vi "Rotation stage shgv3.vi"() -> ()   [LabVIEW 2020]
doc: "Shows how to move a motor to an absolute position."
uses:
  <vilib>/Utility/error.llb/DialogType.ctl
  <vilib>/DAQmx/read.llb/DAQmx Read (Analog 1D Wfm NChan 1Samp).vi
  <vilib>/DAQmx/read.llb/DAQmx Read (Counter 1D U32 1Chan NSamp).vi
  <vilib>/DAQmx/create/channels.llb/DAQmx Create Channel (CI-Period).vi
  <vilib>/DAQmx/create/channels.llb/DAQmx Create Channel (CO-Pulse Generation-Frequency).vi
  <vilib>/DAQmx/configure/timing.llb/DAQmx Timing (Implicit).vi
  <vilib>/DAQmx/miscellaneous.llb/DAQmx Fill In Error Info.vi
  <vilib>/DAQmx/create/channels.llb/DAQmx Create Channel (AI-Current-Basic).vi
  <vilib>/DAQmx/configure/timing.llb/DAQmx Timing (Sample Clock).vi
  <resource>/objmgr/daqmx.rc
panel:
  out "Actual Sample Rate":dbl=1000.0 format="%0.2f"
  out "data 2":waveform(dbl)[](graph)
  out "Consumer Iteration 3":i32=1109257
  in  "stop 4":bool
  out "Producer Iteration 3":i32=1109256
  out "error out 3":errorcluster
  out "Loop Time (ms) 3":u32=10
  in  "Duty Cycle":dbl=0.5 format="%.6f"
  out "Input.BufSize":u32=1000000 format="%.0p"
  out "data":u32[](graph)
  out "Consumer Iteration 2":i32=1109257
  in  "stop 3":bool
  in  "number of samples per channel 2":i32=5000
  out "Producer Iteration 2":i32=1109256
  out "error out 2":errorcluster
  out "Loop Time (ms) 2":u32=10
  in  "dwell time (ms)":dbl=1.0 format="%.6f"
  in  "Photon Input (PFI)":tag="/Dev1/PFI0"
  in  "Rotation Angle (Degrees)":dbl=100.0 min=0.0
  in  "MG17Motor":refnum<k7>(container)
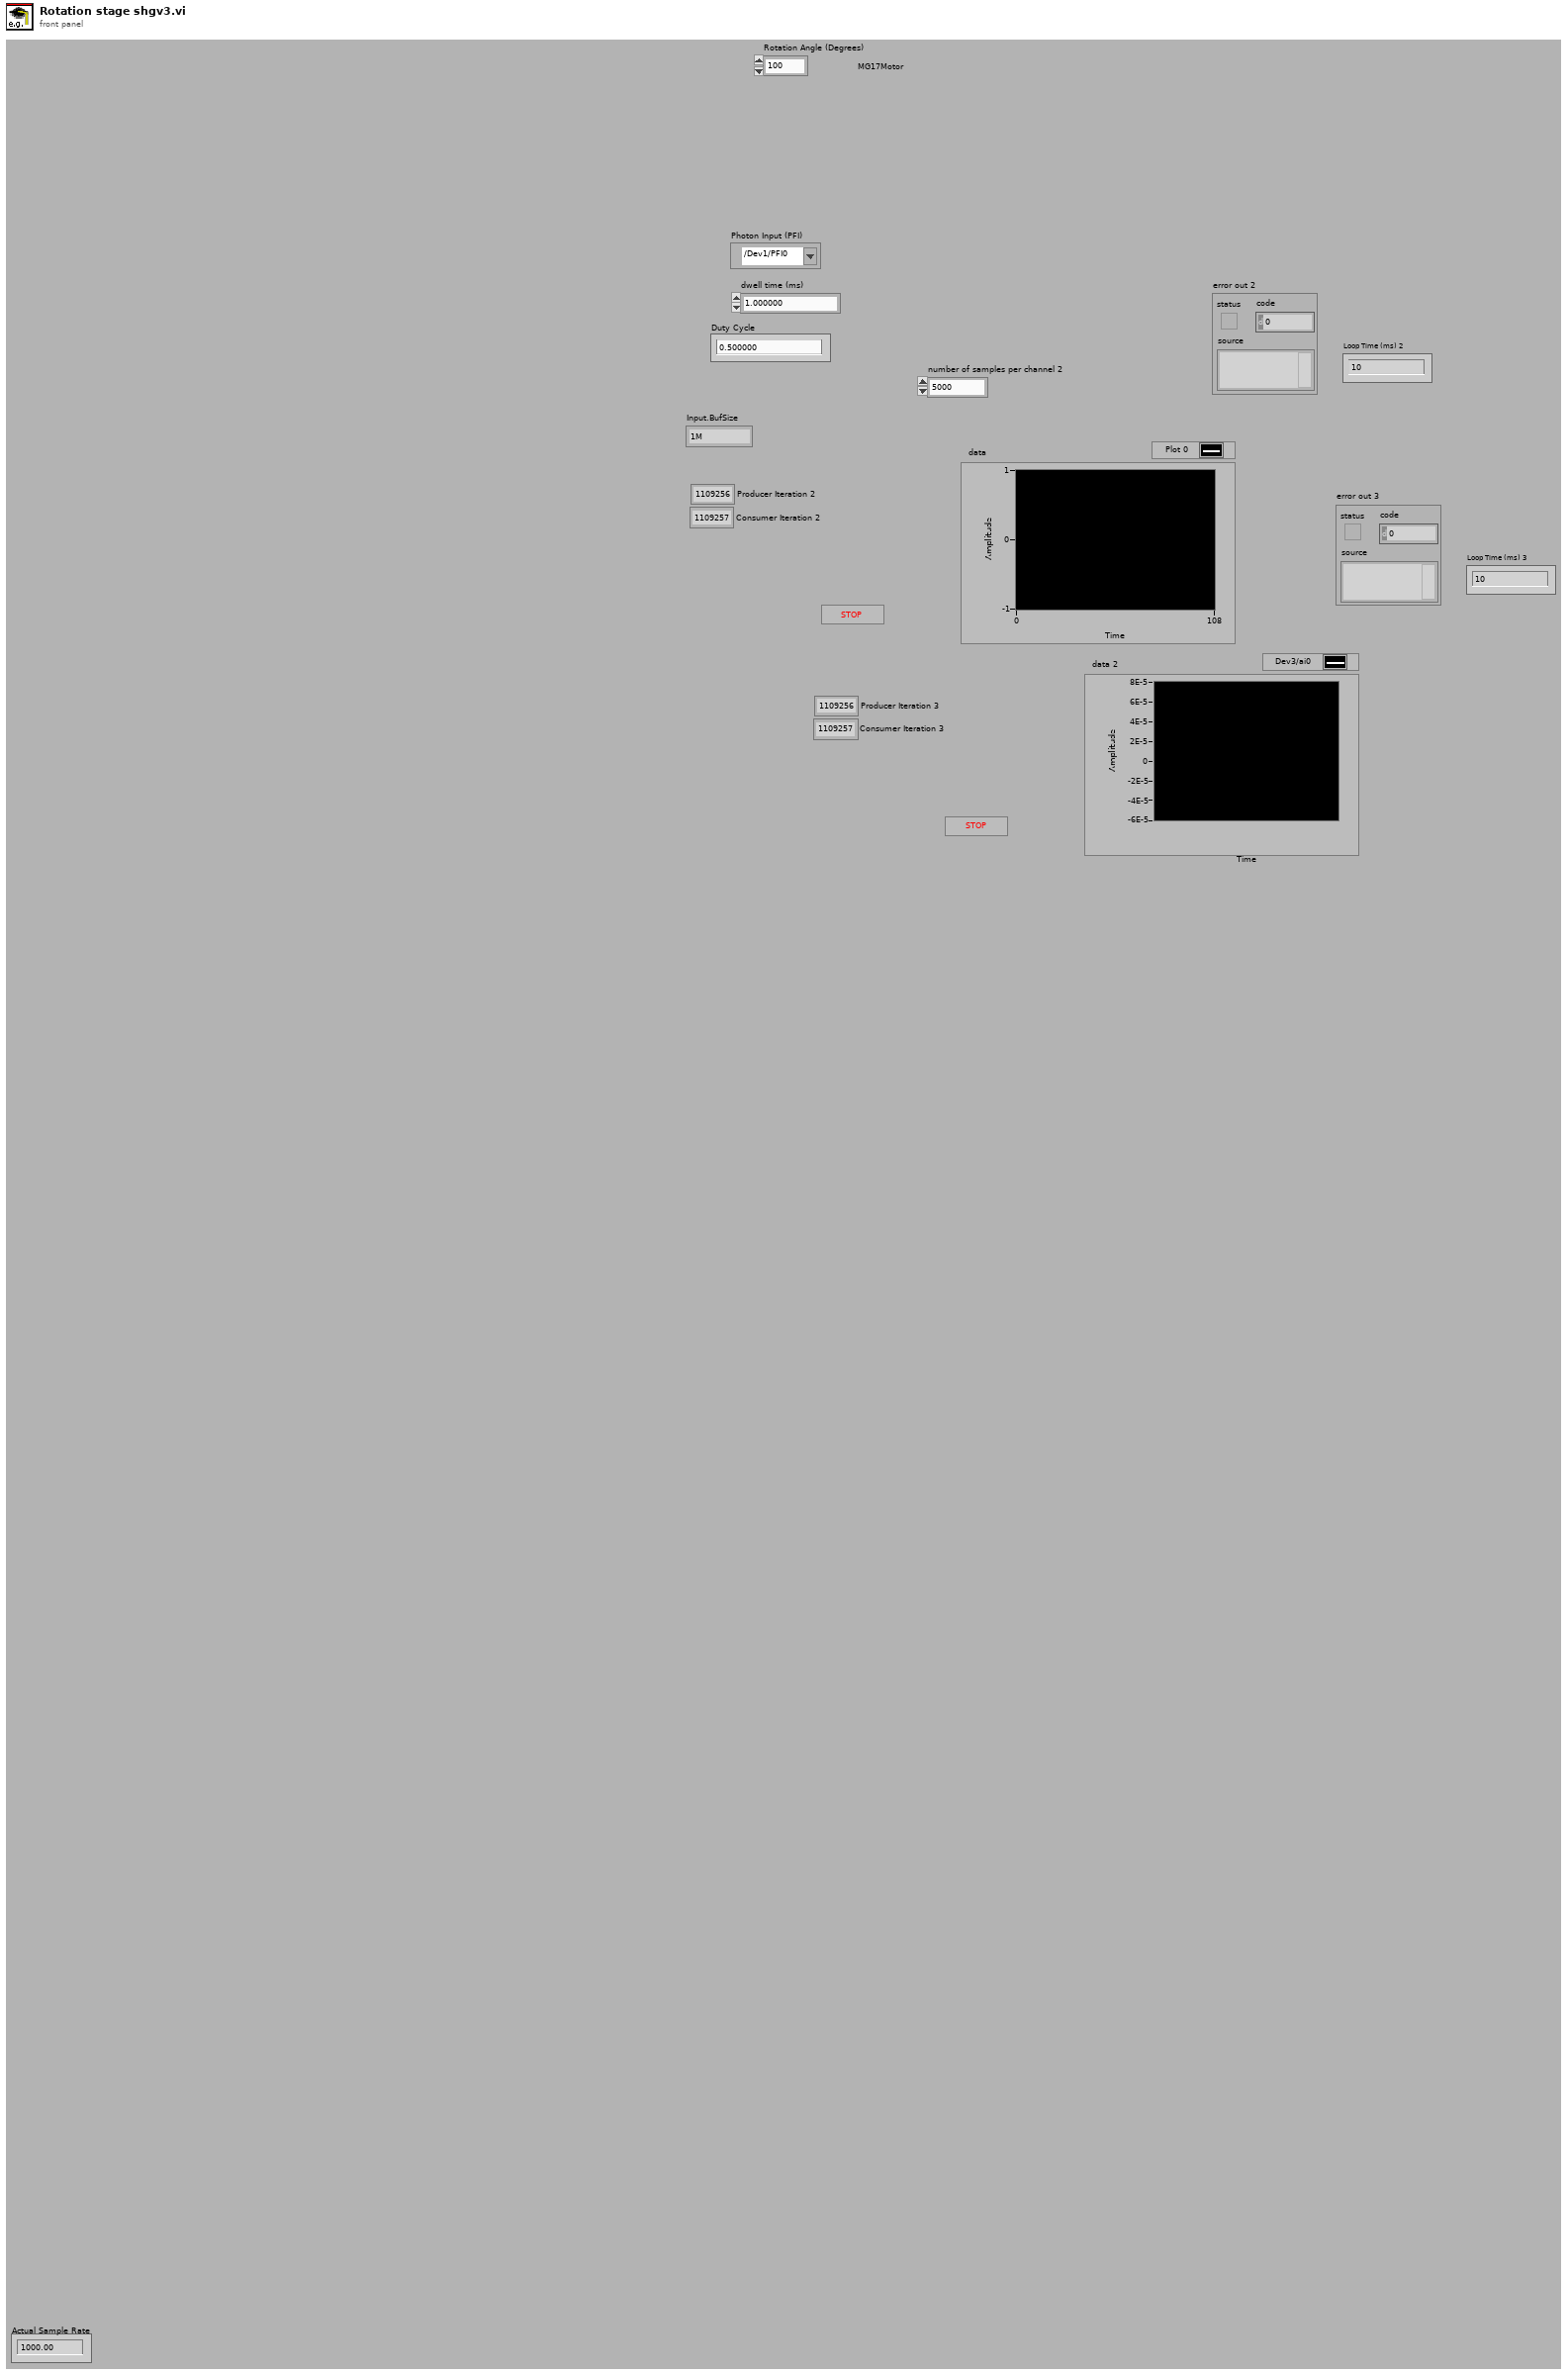
[diagram p1: front panel]
types:
  T1 = enum16{"open", "open or create", "create or replace", "create", "open (read-only)"}
  T2 = typedef "DialogType.ctl" = u16
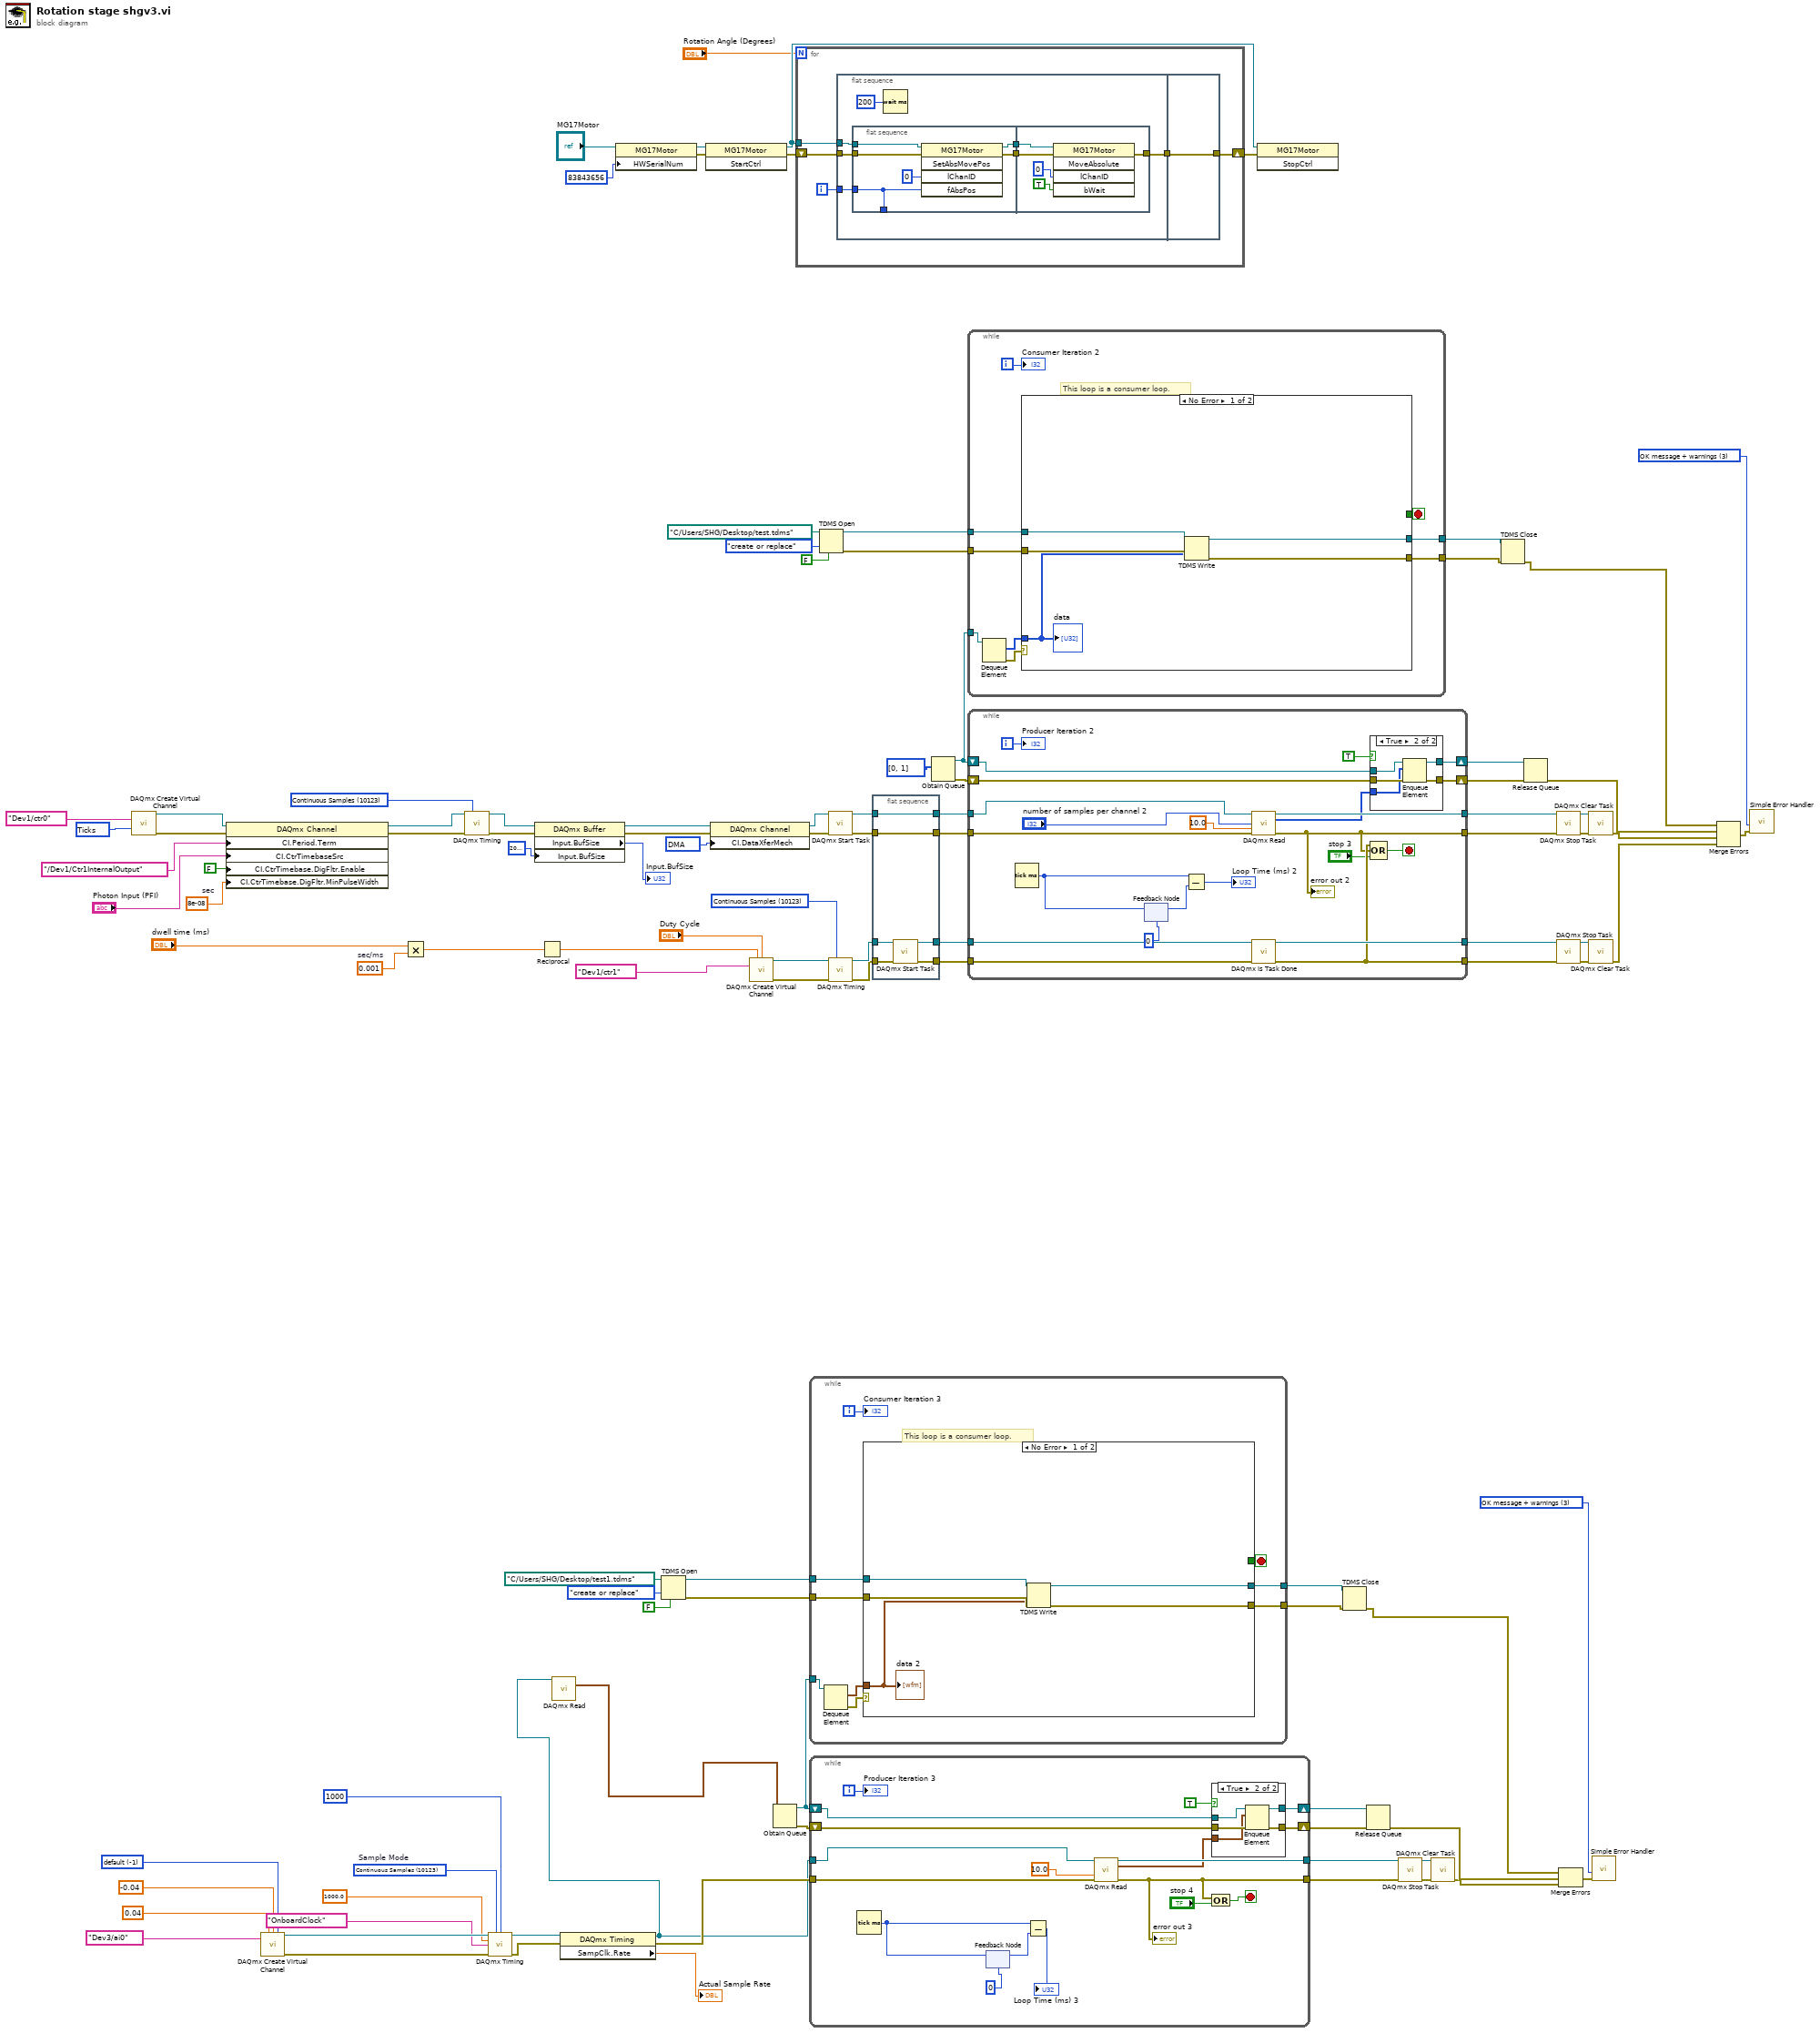
[diagram p0: block diagram]
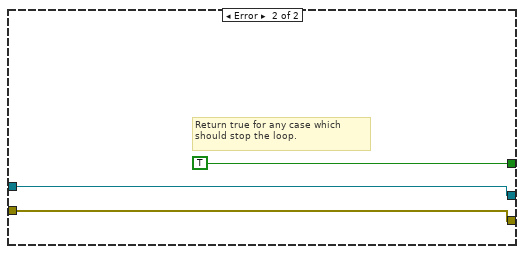
[diagram p2: hidden frame]
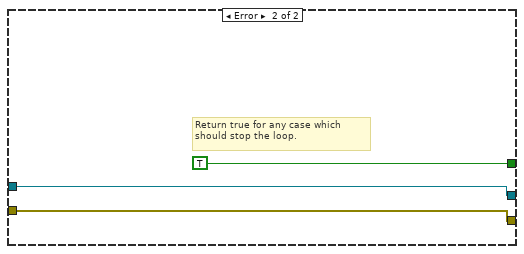
[diagram p4: hidden frame]
diagram:
  w6 = -1 items=["default"=-1, "RSE"=10083, "NRSE"=10078, "Differential"=10106, "Pseudodifferential"=12529] ("Terminal Configuration")
  w14 = 10123 items=["Finite Samples"=10178, "Continuous Samples"=10123, "Hardware Timed Single Point"=12522]  # Sample Mode
  w24 = T2 3 items=["no dialog", "OK message", "continue or stop message", "OK message + warnings", "continue/stop + warnings"] ("type of dialog (OK msg:1)")
  w45 = T2 3 items=["no dialog", "OK message", "continue or stop message", "OK message + warnings", "continue/stop + warnings"] ("type of dialog (OK msg:1)")
  w50 = 8e-08  # sec
  w61 = 10054 items=["DMA"=10054, "Interrupts"=10204, "Programmed I/O"=10264, "USB Bulk"=12590] ("CI.DataXferMech")
  w81 = 0.001  # sec/ms
  w91 = 10304 items=["Seconds"=10364, "Ticks"=10304, "From Custom Scale"=10065] ("units")
  w92 = 10123 items=["Finite Samples"=10178, "Continuous Samples"=10123, "Hardware Timed Single Point"=12522] ("sample mode")
  w93 = 10123 items=["Finite Samples"=10178, "Continuous Samples"=10123, "Hardware Timed Single Point"=12522] ("sample mode")
  n1 = call-poly <vilib>:"DAQmx Create Virtual Channel.vi"("counter"=tag "Dev1/ctr0", "units"=w91) -> ("task out"=w88:refnum<k21>, "error out"=w87:errorcluster)  [unwired: 12 in]
  n2 = property class="DAQmx Channel"(reference=w88, error in=w87, "CI.Period.Term"=tag "/Dev1/Ctr1InternalOutput", "CI.CtrTimebaseSrc"="Photon Input (PFI)", "CI.CtrTimebase.DigFltr.Enable"=FALSE, "CI.CtrTimebase.DigFltr.MinPulseWidth"=w50) -> (reference out=w86:refnum<k21>, error out=w85:errorcluster)
  n3 = call-poly <vilib>:"DAQmx Create Virtual Channel.vi"("maximum value"=0.04 ("Max Voltage"), "minimum value"=-0.04 ("Min Voltage"), "input terminal configuration"=w6, "physical channels"=tag "Dev3/ai0" ("Physical Channel")) -> ("task out"=w12:refnum<k21>, "error out"=w13:errorcluster)  [unwired: 10 in]
  n4 = Multiply(x="dwell time (ms)", y=w81) -> (x*y=w80:dbl)
  n5 = call-poly <vilib>:"DAQmx Timing.vi"("task/channels in"=w86, "sample mode"=w92, "error in"=w85) -> ("task out"=w56:refnum<k21>, "error out"=w55:errorcluster)  [unwired: 11 in]
  n6 = call-poly <vilib>:"DAQmx Timing.vi"("task/channels in"=w12, "sample mode"=w14, "samples per channel"=1000 ("Number of Samples"), "rate"=1000.0 ("Sample Rate"), "source"=tag "OnboardClock" ("Sample Clock Source"), "error in"=w13) -> ("task out"=w16:refnum<k21>, "error out"=w15:errorcluster)  [unwired: 8 in]
  n7 = property class="DAQmx Buffer"(reference=w56, error in=w55, "Input.BufSize"=u32 2000000 ("samples per channel")) -> (reference out=w60:refnum<k21>, error out=w58:errorcluster, "Input.BufSize"=→"Input.BufSize":u32)
  n8 = Reciprocal(x=w80) -> (1/x=w79:dbl)
  n9 = property class="DAQmx Timing"(reference=w16, error in=w15) -> (reference out=w1:refnum<k21>, error out=w10:errorcluster, "SampClk.Rate"=→"Actual Sample Rate":dbl)
  n10 = call-poly <vilib>:"DAQmx Read.vi"("task/channels in"=w1) -> ("data"=w2:waveform(dbl)[])  [unwired: 12 in, 2 out]
  n11 = property class="MG17Motor"(reference="MG17Motor", "HWSerialNum"=83843656) -> (reference out=w103:refnum<k7>, error out=w102:errorcluster)  [unwired: 1 in]
  n12 = TDMS Open(6:FALSE ("disable buffering? (T)"), 10:T1."create or replace" ("operation (0:open)"), 11:path "C:/Users/SHG/Desktop/test1.tdms" ("file path")) -> (0:w26:errorcluster, 3:w28:refnum<k34>)  [unwired: 4 in]
  n13 = invoke class="MG17Motor" method="StartCtrl"(reference=w103, error in=w102) -> (reference out=w107:refnum<k7>, error out=w106:errorcluster)  [unwired: 1 in, 1 out]
  n14 = property class="DAQmx Channel"(reference=w60, error in=w58, "CI.DataXferMech"=w61) -> (reference out=w54:refnum<k21>, error out=w53:errorcluster)
  n15 = call-poly <vilib>:"DAQmx Create Virtual Channel.vi"("frequency"=w79, "duty cycle"="Duty Cycle", "counter"=tag "Dev1/ctr1") -> ("task out"=w98:refnum<k21>, "error out"=w99:errorcluster)  [unwired: 11 in]
  n16 = Obtain Queue(element data type=w2) -> (queue out=w36:refnum<queue>, error out=w35:errorcluster)  [unwired: 4 in, 1 out]
  n17 = for {
    N: "Rotation Angle (Degrees)" -> [_]
    tunnel: w107 -> [w112]
    shift-right: [w110] -> w105
    shift-left: w106 -> [w111]
    i -> [w108]
    n18 = flat-sequence {
      tunnel: w112 -> [w117]
      tunnel: w111 -> [w115]
      tunnel: [w114] -> w109
      tunnel: w108 -> [w116]
      tunnel: [w131] -> w110
      tunnel: w109 -> [w131]
      frame #0 {
        n19 = flat-sequence {
          tunnel: [w120] -> _
          tunnel: w115 -> [w124]
          tunnel: w117 -> [w123]
          tunnel: [w122] -> w119
          tunnel: [w121] -> w118
          tunnel: w116 -> [w120]
          tunnel: w119 -> [w128]
          tunnel: w118 -> [w127]
          tunnel: [w126] -> w114
          frame #0 {
            n20 = invoke class="MG17Motor" method="SetAbsMovePos"(reference=w123, error in=w124, "lChanID"=0, "fAbsPos"=w120) -> (reference out=w121:refnum<k7>, error out=w122:errorcluster)  [unwired: 1 in, 3 out]
          }
          frame #1 {
            n21 = invoke class="MG17Motor" method="MoveAbsolute"(reference=w127, error in=w128, "lChanID"=0, "bWait"=TRUE) -> (error out=w126:errorcluster)  [unwired: 1 in, 4 out]
          }
        }
        n22 = Wait (ms)(milliseconds to wait=u32 200) -> ()  [unwired: 1 out]
      }
      frame #1 {
      }
    }
  }
  n23 = while {
    tunnel: w36 -> [w140]
    tunnel: w28 -> [w135]
    tunnel: [w134] -> w27
    tunnel: w26 -> [w133]
    tunnel: [w132] -> w25
    i -> [w136]
    stop <- w137 stop-if-true
    # "This loop is a consumer loop."
    n24 = Dequeue Element(queue=w140) -> (element=w138:waveform(dbl)[], error out=w139:errorcluster)  [unwired: 2 in, 2 out]
    n25 = case shown="No Error" w139 {
      tunnel: w138 -> [w141 _]
      tunnel: [_ TRUE] -> w137
      tunnel: w135 -> [w145 w147]
      tunnel: [w144 w147] -> w134
      tunnel: w133 -> [w143 w146]
      tunnel: [w142 w146] -> w132
      frame No Error {
        n26 = TDMS Write(0:w145, 9:w141, 11:w143) -> (4:w144:refnum<k34>, 15:w142:errorcluster)  [unwired: 3 in, 2 out]
        "data 2" <- w141
      }
      frame Error {
        # "Return true for any case which should stop the loop."
      }
    }
    "Consumer Iteration 3" <- w136
  }
  n27 = while {
    shift-right: [w156] -> w33
    shift-left: w35 -> [w164]
    shift-right: [w165] -> w34
    shift-left: w36 -> [w166]
    tunnel: [w162] -> w30
    tunnel: [w155] -> w29
    tunnel: w10 -> [w161]
    tunnel: w1 -> [w160]
    i -> [w157]
    stop <- w153 stop-if-true
    n28 = Tick Count (ms)() -> (millisecond timer value=w152:u32)
    n29 = feedback #1(u32 0 ("millisecond timer value")) -> (w151:u32)
    n30 = feedback-in #1(w152) -> ()
    n31 = Subtract(x=w152, y=w151) -> (x-y=→"Loop Time (ms) 3":u32)
    n32 = call-poly <vilib>:"DAQmx Read.vi"("task/channels in"=w160, "timeout"=10.0, "error in"=w161) -> ("task out"=w162:refnum<k21>, "data"=w159:waveform(dbl)[], "error out"=w155:errorcluster)  [unwired: 10 in]
    "error out 3" <- w155
    n33 = case shown="True" TRUE ("Case Constant\n(See Context Help)") {
      tunnel: w166 -> [w168 w173]
      tunnel: [w168 w172] -> w165
      tunnel: w164 -> [w167 w171]
      tunnel: [w167 w170] -> w156
      tunnel: w159 -> [_ w169]
      frame False {
      }
      frame True {
        n34 = Enqueue Element(queue=w173, element=w169, error in (no error)=w171) -> (queue out=w172:refnum<queue>, error out=w170:errorcluster)  [unwired: 1 in, 1 out]
      }
    }
    n35 = Compound Arithmetic op=OR(w155, "stop 4") -> (w153:bool)
    "Producer Iteration 3" <- w157
  }
  n36 = TDMS Open(6:FALSE ("disable buffering? (T)"), 10:T1."create or replace" ("operation (0:open)"), 11:path "C:/Users/SHG/Desktop/test.tdms" ("file path")) -> (0:w47:errorcluster, 3:w49:refnum<k34>)  [unwired: 4 in]
  n37 = call <vilib>:"DAQmx Start Task.vi"("task/channels in"=w54, "error in"=w53) -> ("task out"=w78:refnum<k21>, "error out"=w77:errorcluster)  [unwired: 12 in]
  n38 = call-poly <vilib>:"DAQmx Timing.vi"("task/channels in"=w98, "sample mode"=w93, "error in"=w99) -> ("task out"=w97:refnum<k21>, "error out"=w96:errorcluster)  [unwired: 11 in]
  n39 = flat-sequence {
    tunnel: w97 -> [w179]
    tunnel: w96 -> [w178]
    tunnel: [w177] -> w64
    tunnel: [w176] -> w65
    tunnel: w78 -> [w174]
    tunnel: w77 -> [w175]
    tunnel: [w175] -> w67
    tunnel: [w174] -> w66
    frame #0 {
      n40 = call <vilib>:"DAQmx Start Task.vi"("task/channels in"=w179, "error in"=w178) -> ("task out"=w176:refnum<k21>, "error out"=w177:errorcluster)  [unwired: 12 in]
    }
  }
  n41 = Obtain Queue(element data type=u32[] [0, 1] ("data")) -> (queue out=w76:refnum<queue>, error out=w75:errorcluster)  [unwired: 4 in, 1 out]
  n42 = while {
    tunnel: w76 -> [w188]
    tunnel: w49 -> [w183]
    tunnel: [w182] -> w48
    tunnel: w47 -> [w181]
    tunnel: [w180] -> w46
    i -> [w184]
    stop <- w185 stop-if-true
    # "This loop is a consumer loop."
    n43 = Dequeue Element(queue=w188) -> (element=w186:u32[], error out=w187:errorcluster)  [unwired: 2 in, 2 out]
    n44 = case shown="No Error" w187 {
      tunnel: w186 -> [w189 _]
      tunnel: [_ TRUE] -> w185
      tunnel: w183 -> [w193 w195]
      tunnel: [w192 w195] -> w182
      tunnel: w181 -> [w191 w194]
      tunnel: [w190 w194] -> w180
      frame No Error {
        n45 = TDMS Write(0:w193, 9:w189, 11:w191) -> (4:w192:refnum<k34>, 15:w190:errorcluster)  [unwired: 3 in, 2 out]
        "data" <- w189
      }
      frame Error {
        # "Return true for any case which should stop the loop."
      }
    }
    "Consumer Iteration 2" <- w184
  }
  n46 = while {
    shift-right: [w208] -> w73
    shift-left: w75 -> [w217]
    shift-right: [w218] -> w74
    shift-left: w76 -> [w219]
    tunnel: [w215] -> w70
    tunnel: [w203] -> w69
    tunnel: w67 -> [w214]
    tunnel: w66 -> [w213]
    tunnel: w65 -> [w207]
    tunnel: w64 -> [w206]
    tunnel: [w205] -> w63
    tunnel: [w204] -> w62
    i -> [w209]
    stop <- w201 stop-if-true
    n47 = Tick Count (ms)() -> (millisecond timer value=w200:u32)
    n48 = feedback #2(u32 0 ("millisecond timer value")) -> (w199:u32)
    n49 = feedback-in #2(w200) -> ()
    n50 = Subtract(x=w200, y=w199) -> (x-y=→"Loop Time (ms) 2":u32)
    n51 = call-poly <vilib>:"DAQmx Read.vi"("task/channels in"=w213, "number of samples per channel"="number of samples per channel 2", "timeout"=10.0, "error in"=w214) -> ("task out"=w215:refnum<k21>, "data"=w212:u32[], "error out"=w203:errorcluster)  [unwired: 9 in]
    "error out 2" <- w203
    n52 = call <vilib>:"DAQmx Is Task Done.vi"("task/channels in"=w207, "error in"=w206) -> ("task out"=w205:refnum<k21>, "error out"=w204:errorcluster)  [unwired: 11 in, 1 out]
    n53 = case shown="True" TRUE ("Case Constant\n(See Context Help)") {
      tunnel: w219 -> [w221 w226]
      tunnel: [w221 w225] -> w218
      tunnel: w217 -> [w220 w224]
      tunnel: [w220 w223] -> w208
      tunnel: w212 -> [_ w222]
      frame False {
      }
      frame True {
        n54 = Enqueue Element(queue=w226, element=w222, error in (no error)=w224) -> (queue out=w225:refnum<queue>, error out=w223:errorcluster)  [unwired: 1 in, 1 out]
      }
    }
    n55 = Compound Arithmetic op=OR(w204, w203, "stop 3") -> (w201:bool)
    "Producer Iteration 2" <- w209
  }
  n56 = invoke class="MG17Motor" method="StopCtrl"(reference=w107, error in=w105) -> ()  [unwired: 1 in, 3 out]
  n57 = TDMS Close(8:w25, 11:w27) -> (0:w20:errorcluster)  [unwired: 1 out]
  n58 = Release Queue(queue=w34, error in (no error)=w33) -> (error out=w19:errorcluster)  [unwired: 1 in, 2 out]
  n59 = call <vilib>:"DAQmx Stop Task.vi"("task/channels in"=w30, "error in"=w29) -> ("task out"=w31:refnum<k21>, "error out"=w32:errorcluster)  [unwired: 12 in]
  n60 = call <vilib>:"DAQmx Clear Task.vi"("task in"=w31, "error in"=w32) -> ("error out"=w18:errorcluster)  [unwired: 13 in]
  n61 = TDMS Close(8:w46, 11:w48) -> (0:w41:errorcluster)  [unwired: 1 out]
  n62 = Release Queue(queue=w74, error in (no error)=w73) -> (error out=w40:errorcluster)  [unwired: 1 in, 2 out]
  n63 = call <vilib>:"DAQmx Stop Task.vi"("task/channels in"=w70, "error in"=w69) -> ("task out"=w71:refnum<k21>, "error out"=w72:errorcluster)  [unwired: 12 in]
  n64 = call <vilib>:"DAQmx Stop Task.vi"("task/channels in"=w63, "error in"=w62) -> ("task out"=w95:refnum<k21>, "error out"=w94:errorcluster)  [unwired: 12 in]
  n65 = Merge Errors(w20, w19, w18) -> (w23:errorcluster)
  n66 = call <vilib>:"DAQmx Clear Task.vi"("task in"=w71, "error in"=w72) -> ("error out"=w39:errorcluster)  [unwired: 13 in]
  n67 = call <vilib>:"DAQmx Clear Task.vi"("task in"=w95, "error in"=w94) -> ("error out"=w38:errorcluster)  [unwired: 13 in]
  n68 = call <vilib>:"Simple Error Handler.vi"("type of dialog (OK msg:1)"=w24, "error in (no error)"=w23) -> ()  [unwired: 3 in, 5 out]
  n69 = Merge Errors(w41, w40, w39, w38) -> (w44:errorcluster)
  n70 = call <vilib>:"Simple Error Handler.vi"("type of dialog (OK msg:1)"=w45, "error in (no error)"=w44) -> ()  [unwired: 3 in, 5 out]
